vi "Unreserve Hardware for DAQmx Task.vi"(8 "error in (no error)":errorcluster, 11 "task/channels in":refnum<k21>) -> (0 "error out":errorcluster, 3 "task out":refnum<k21>)   [LabVIEW 2015, in "PL Utility.lvlib"]
doc: "Unreserves the hardware resources needed for the DAQmx task."
uses:
  PL Utility.lvlib
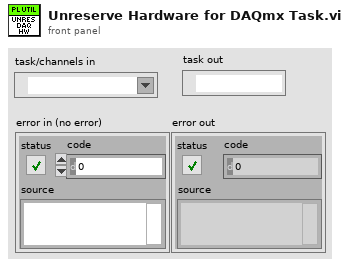
[diagram p1: front panel]
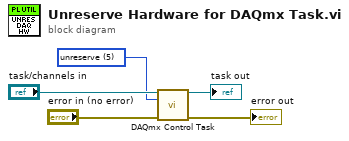
[diagram p0: block diagram]
diagram:
  w1 = 5 items=["verify"=2, "reserve"=4, "commit"=3, "unreserve"=5, "abort"=6] ("action")
  n1 = call <vilib>:"DAQmx Control Task.vi"("task/channels in"="task/channels in", "action"=w1, "error in"="error in (no error)") -> ("task out"=→"task out":refnum<k21>, "error out"=→"error out":errorcluster)  [unwired: 11 in]
